vi "Program Stop.vi"(3 "user event":refnum<user-event>, 5 "Event Registration Refnum in":refnum<event-registration>, 6 "GUI queue":refnum<queue>, 7 "control queue":refnum<queue>, 8 "operation queue":refnum<queue>, 9 "GUI error":errorcluster, 10 "operation error":errorcluster, 11 "control error":errorcluster) -> ()   [LabVIEW 2011]
uses:
  Controls/User Interface Control.ctl
  Controls/User Interface Action.ctl
  Controls/User Event Control.ctl
  Controls/User Event Action.ctl
  Error Handling/Error Module Action.ctl
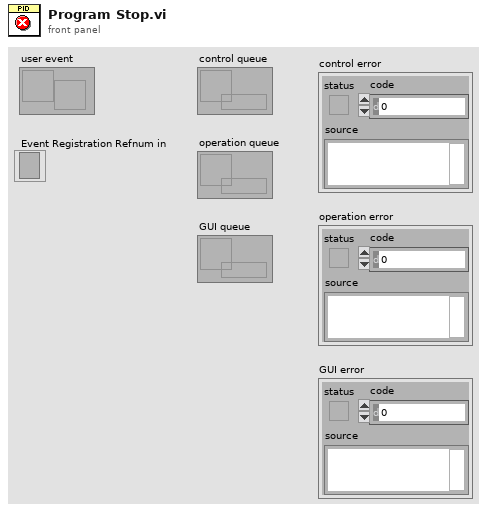
[diagram p1: front panel]
types:
  T1 = typedef "Error Module Action.ctl" = enum16{"Initialize", "Handle Errors", "Report Errors"}
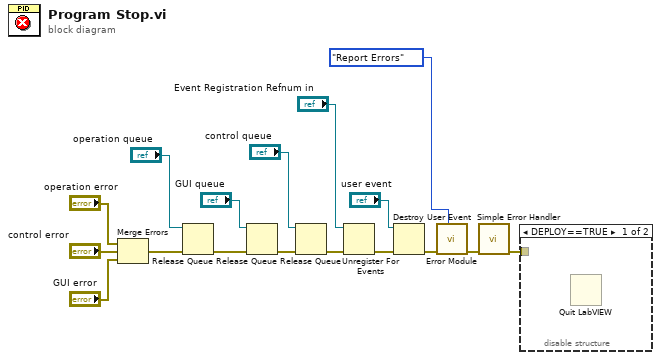
[diagram p0: block diagram]
diagram:
  n1 = Merge Errors("operation error", "control error", "GUI error") -> (w10:errorcluster)
  n2 = Release Queue(queue="operation queue", error in (no error)=w10) -> (error out=w11:errorcluster)  [unwired: 1 in, 2 out]
  n3 = Release Queue(queue="GUI queue", error in (no error)=w11) -> (error out=w3:errorcluster)  [unwired: 1 in, 2 out]
  n4 = Release Queue(queue="control queue", error in (no error)=w3) -> (error out=w2:errorcluster)  [unwired: 1 in, 2 out]
  n5 = Unregister For Events(event registration refnum="Event Registration Refnum in", error in=w2) -> (error out=w12:errorcluster)
  n6 = Destroy User Event(user event="user event", error in=w12) -> (error out=w14:errorcluster)
  n7 = call "Error Module.vi"("Command (Handle Errors"=Error_Module_Action."Report Errors", "error in"=w14) -> ("error out"=w15:errorcluster)  [unwired: 8 in, 1 out]
  n8 = call <vilib>:"Simple Error Handler.vi"("error in (no error)"=w15) -> ("error out"=w16:errorcluster)  [unwired: 4 in, 4 out]
  n9 = disable-structure shown="DEPLOY==TRUE" {
    disable-tunnel: w16 -> [_ _]
    frame condition #0 {
      n10 = Quit LabVIEW() -> ()  [unwired: 1 in]
    }
    frame condition #1 (active) {
    }
  }
